vi "myfirst4.vi"() -> ()   [LabVIEW 2020]
panel:
  out "Array 6":bool[](array[boolean])
  out "Array 5":string[](array[string])
  out "Array 4":dbl[](array[numeric])
  in  "Array 3":bool[](array[boolean])
  in  "Array 2":string[](array[string])
  in  "Array":dbl[](array[numeric])
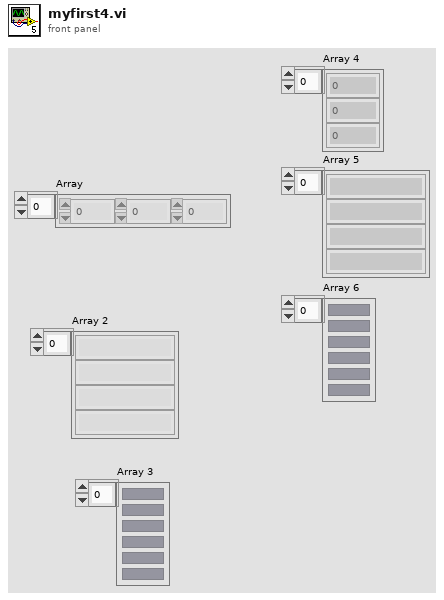
[diagram p1: front panel]
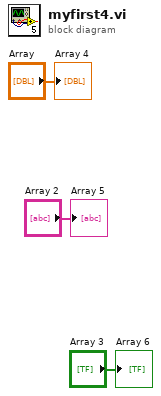
[diagram p0: block diagram]
diagram:
  "Array 4" <- "Array"
  "Array 5" <- "Array 2"
  "Array 6" <- "Array 3"
